vi "Delete Insert Test.vi"() -> ()   [LabVIEW 2015]
uses:
  Insert into Object.vi
  JSONtext.lvlib
panel:
  out "Array 2":string[](array[string])
  out "Passed":bool[](array[boolean])
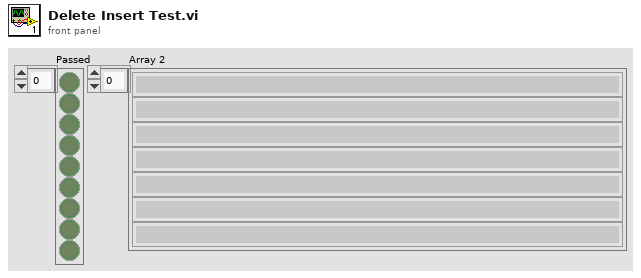
[diagram p1: front panel]
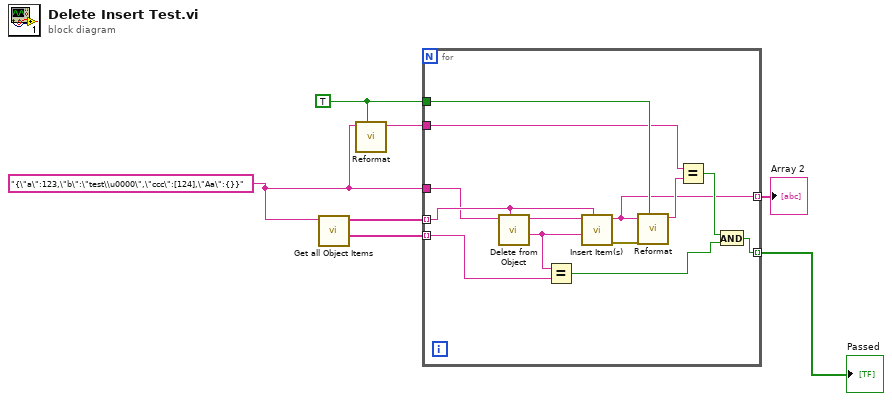
[diagram p0: block diagram]
diagram:
  w3 = TRUE ("Alphabetical Sort Objects")
  w4 = "{\"a\":123,\"b\":\"test\\u0000\",\"ccc\":[124],\"Aa\":{}}"
  n1 = call "Get all Object Items.vi"("JSON"=w4) -> ("<JSON>"=w7:string[], "Names"=w6:string[])  [unwired: 7 in, 2 out]
  n2 = call "Reformat.vi"("Alphabetical Sort Objects"=w3, "Input String"=w4) -> ("<JSON>First JSON Value"=w2:string)  [unwired: 6 in, 3 out]
  n3 = for {
    tunnel: w4 -> [w17]
    tunnel: w7 -> [w18] mode=indexing
    tunnel: w6 -> [w20] mode=indexing
    tunnel: [w9] -> w5 mode=indexing
    tunnel: w3 -> [w14]
    tunnel: w2 -> [w12]
    tunnel: [w8] -> w1 mode=indexing
    n4 = call "Delete from Object.vi"("Object (or Item) Path"=w20, "JSON in"=w17) -> ("<JSON>Deleted"=w16:string, "<JSON>"=w19:string)  [unwired: 5 in, 2 out]
    n5 = Equal?(x=w16, y=w18) -> (x = y?=w11:bool)
    n6 = call-poly "Insert Item(s).vi"("Object (or Item) Path"=w20, "JSON to Insert"=w16, "JSON in"=w19) -> ("error out"=w15:errorcluster, "<JSON>"=w8:string)  [unwired: 5 in, 1 out]
    n7 = call "Reformat.vi"("Alphabetical Sort Objects"=w14, "error in (no error)"=w15, "Input String"=w8) -> ("<JSON>First JSON Value"=w13:string)  [unwired: 5 in, 3 out]
    n8 = Equal?(x=w12, y=w13) -> (x = y?=w10:bool)
    n9 = And(x=w10, y=w11) -> (x .and. y?=w9:bool)
  }
  "Passed" <- w5
  "Array 2" <- w1
